vi "Reset.vi"(8 "error in":errorcluster, 11 "5745A in":refnum<class "5745A.lvclass">) -> (0 "error out":errorcluster, 3 "5745A out":refnum<class "5745A.lvclass">)   [LabVIEW 2018, in "5745A.lvlib" / "5745A.lvclass"]
uses:
  5745A.lvclass
  builds/Power_Supply.lvlibp/Power Supply.lvclass
  C:/Users/Ron.Dexter.LUMINARTECH/Desktop/builds/Power_Supply.lvlibp/Power Supply.lvclass
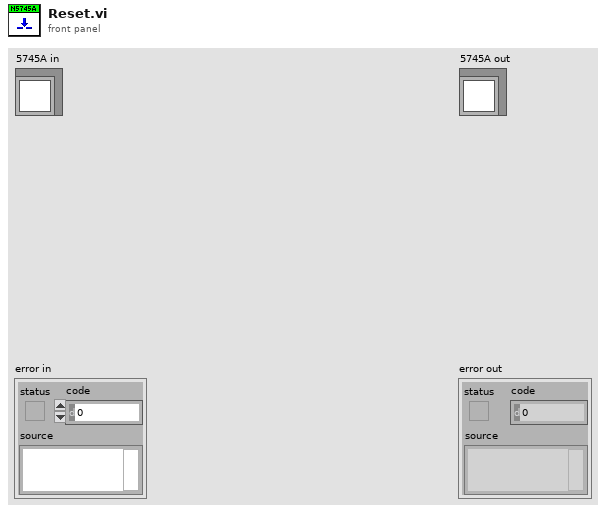
[diagram p1: front panel]
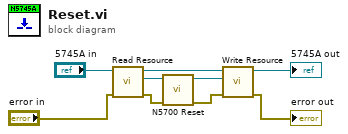
[diagram p0: block diagram]
diagram:
  n1 = call "Read Resource.vi"("error in"="error in", "Power Supply in"="5745A in") -> ("error out"=w6:errorcluster, "Resource"=w7:refnum<visa-resource-name>, "Power Supply out"=w2:refnum<class "5745A.lvclass">)  [unwired: 7 in]
  n2 = call <instrlib>:"N5700 Reset.vi"("error"=w6, "VISA"=w7) -> ("error out"=w4:errorcluster, "VISA out"=w5:refnum<visa-resource-name>)  [unwired: 5 in]
  n3 = call "Write Resource.vi"("error in"=w4, "Resource"=w5, "Power Supply in"=w2) -> ("error out"=→"error out":errorcluster, "Power Supply out"=→"5745A out":refnum<class "5745A.lvclass">)  [unwired: 7 in]
